vi "Picometer Control.vi"(0 "Cmd":u8 format="%.0x", 5 "ulValue":u32, 7 "uLPtr":u32[](array[numeric]), 9 "BytePtr":u8[](array[numeric]), 11 "error in (no error)":errorcluster) -> (4 "function return":string, 6 "ulValue":u32, 8 "uLPtr":u32[](array[numeric]), 10 "BytePtr":u8[](array[numeric]), 15 "error out":errorcluster)   [LabVIEW 2017, in "ZBOX_IS.lvlib"]
doc: "char *PicometerControl(\n unsigned char Cmd, unsigned long ulValue, unsigned long *uLPtr, unsigned char *BytePtr );"
uses:
  ZBOX_IS.lvlib
  PicometerCtrl.dll
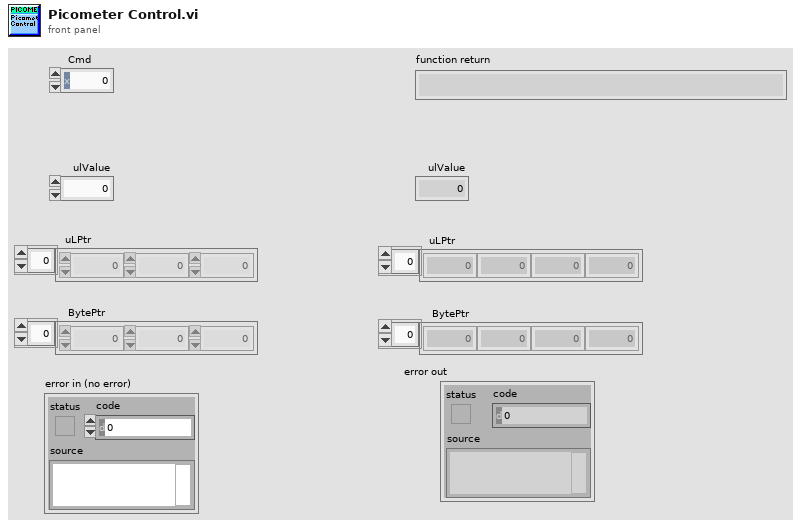
[diagram p1: front panel]
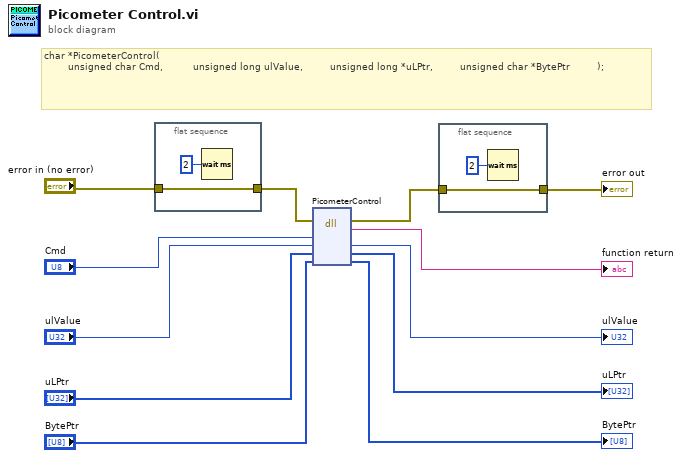
[diagram p0: block diagram]
diagram:
  # "char *PicometerControl(\n\t\t\t\t\t   unsigned char Cmd,\t\t\t\t\t\t\t   unsigned long ulValue,\t\t\t\t\t\t   unsigned long *uLPtr,\t\t\t\t\t\t   unsigned char *BytePtr\t\t\t\t\t\t   );"
  n1 = flat-sequence {
    tunnel: "error in (no error)" -> [w14]
    tunnel: [w14] -> w2
    frame #0 {
      n2 = Wait (ms)(milliseconds to wait=u32 2) -> ()  [unwired: 1 out]
    }
  }
  n3 = dll-call lib="C:/Users/Marek/Desktop/Quadra Software Package v1.1/LabView/Zbox_is/Public/Configure/Low Level/__DLL_functions/PicometerCtrl.dll" fn="PicometerControl"(error in=w2, "Cmd"="Cmd", "ulValue"="ulValue", "uLPtr"="uLPtr", "BytePtr"="BytePtr") -> (error out=w4:errorcluster, "return type"=→"function return":string, "ulValue"=→"ulValue":u32, "uLPtr"=→"uLPtr":u32[], "BytePtr"=→"BytePtr":u8[])  [unwired: 3 in, 1 out]
  n4 = flat-sequence {
    tunnel: w4 -> [w16]
    tunnel: [w16] -> w3
    frame #0 {
      n5 = Wait (ms)(milliseconds to wait=u32 2) -> ()  [unwired: 1 out]
    }
  }
  "error out" <- w3
